vi "Average Corner Coordinates (SubVI).vi"(0 "Raw lcx":dbl, 1 "Raw lcy":dbl, 2 "Raw rcx":dbl, 3 "Raw rcy":dbl, 4 "Input lcx Array":dbl[](array[numeric]), 5 "Input lcy Array":dbl[](array[numeric]), 6 "Input rcx Array":dbl[](array[numeric]), 7 "Input rcy Array":dbl[](array[numeric])) -> (20 "Avg lcx":dbl, 21 "Avg lcy":dbl, 22 "Avg rcx":dbl, 23 "Avg rcy":dbl, 24 "Output lcx Array":dbl[](array[numeric]), 25 "Output lcy Array":dbl[](array[numeric]), 26 "Output rcx Array":dbl[](array[numeric]), 27 "Output rcy Array":dbl[](array[numeric]))   [LabVIEW 2015]
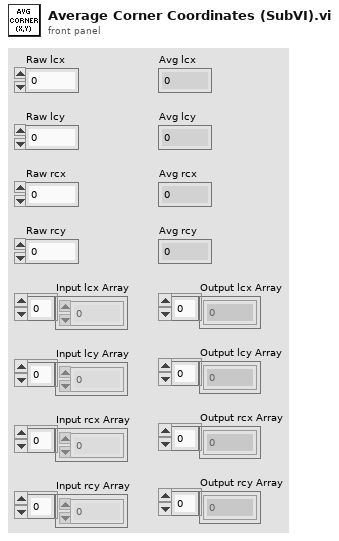
[diagram p1: front panel]
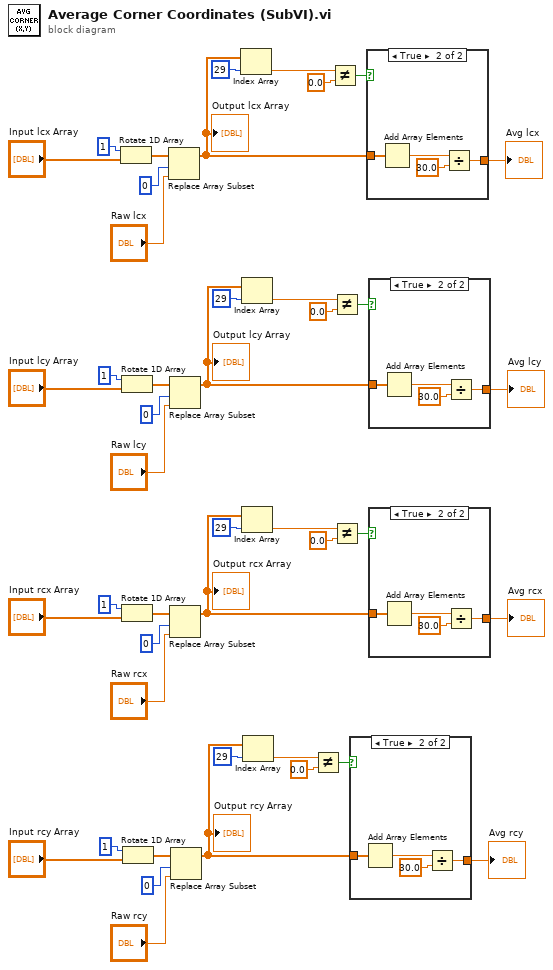
[diagram p0: block diagram]
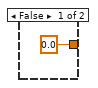
[diagram p2: hidden frame]
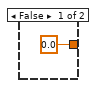
[diagram p3: hidden frame]
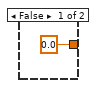
[diagram p4: hidden frame]
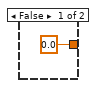
[diagram p5: hidden frame]
diagram:
  n1 = Rotate 1D Array(1:"Input lcx Array", 2:1 ("n")) -> (0:w6:dbl[])
  n2 = Rotate 1D Array(1:"Input lcy Array", 2:1 ("n")) -> (0:w13:dbl[])
  n3 = Rotate 1D Array(1:"Input rcx Array", 2:1 ("n")) -> (0:w20:dbl[])
  n4 = Rotate 1D Array(1:"Input rcy Array", 2:1 ("n")) -> (0:w27:dbl[])
  n5 = Replace Array Subset(array=w6, new element="Raw lcx", index=0) -> (w30:dbl[])
  "Output lcx Array" <- w30
  n6 = Replace Array Subset(array=w13, new element="Raw lcy", index=0) -> (w31:dbl[])
  "Output lcy Array" <- w31
  n7 = Replace Array Subset(array=w20, new element="Raw rcx", index=0) -> (w32:dbl[])
  "Output rcx Array" <- w32
  n8 = Replace Array Subset(array=w27, new element="Raw rcy", index=0) -> (w33:dbl[])
  "Output rcy Array" <- w33
  n9 = Index Array(array=w30, index=29) -> (element=w3:dbl)
  n10 = Index Array(array=w31, index=29) -> (element=w10:dbl)
  n11 = Index Array(array=w32, index=29) -> (element=w17:dbl)
  n12 = Index Array(array=w33, index=29) -> (element=w24:dbl)
  n13 = Not Equal?(x=w24, y=0.0) -> (x != y?=w22:bool)
  n14 = Not Equal?(x=w3, y=0.0) -> (x != y?=w1:bool)
  n15 = Not Equal?(x=w10, y=0.0) -> (x != y?=w8:bool)
  n16 = Not Equal?(x=w17, y=0.0) -> (x != y?=w15:bool)
  n17 = case shown="True" w22 {
    tunnel: w33 -> [_ w49]
    tunnel: [0.0 w46] -> w44
    frame False {
    }
    frame True {
      n18 = Add Array Elements(numeric array=w49) -> (sum=w48:dbl)
      n19 = Divide(x=w48, y=30.0) -> (x/y=w46:dbl)
    }
  }
  "Avg rcy" <- w44
  n20 = case shown="True" w1 {
    tunnel: w30 -> [_ w54]
    tunnel: [0.0 w51] -> w41
    frame False {
    }
    frame True {
      n21 = Add Array Elements(numeric array=w54) -> (sum=w53:dbl)
      n22 = Divide(x=w53, y=30.0) -> (x/y=w51:dbl)
    }
  }
  "Avg lcx" <- w41
  n23 = case shown="True" w8 {
    tunnel: w31 -> [_ w59]
    tunnel: [0.0 w56] -> w42
    frame False {
    }
    frame True {
      n24 = Add Array Elements(numeric array=w59) -> (sum=w58:dbl)
      n25 = Divide(x=w58, y=30.0) -> (x/y=w56:dbl)
    }
  }
  "Avg lcy" <- w42
  n26 = case shown="True" w15 {
    tunnel: w32 -> [_ w64]
    tunnel: [0.0 w61] -> w43
    frame False {
    }
    frame True {
      n27 = Add Array Elements(numeric array=w64) -> (sum=w63:dbl)
      n28 = Divide(x=w63, y=30.0) -> (x/y=w61:dbl)
    }
  }
  "Avg rcx" <- w43
